vi "Check_Ch_Name_colons.vi"(1 "No of Colons":i32, 2 "Ch Name in":string) -> (0 "Ch Name out":string)   [LabVIEW 2018]
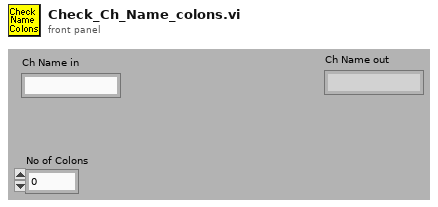
[diagram p1: front panel]
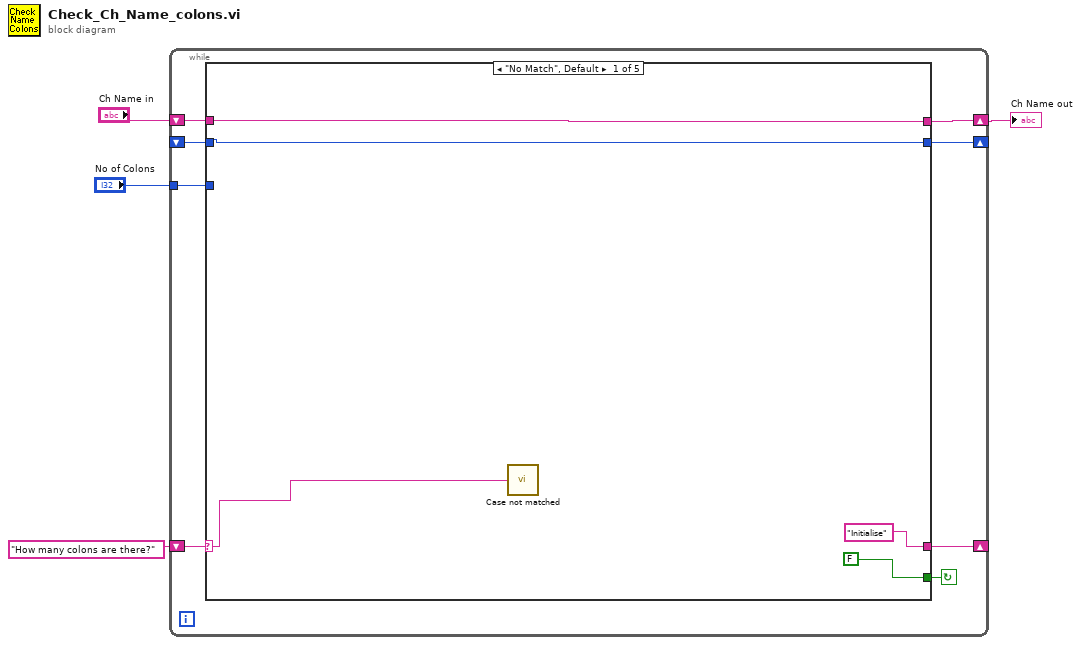
[diagram p0: block diagram]
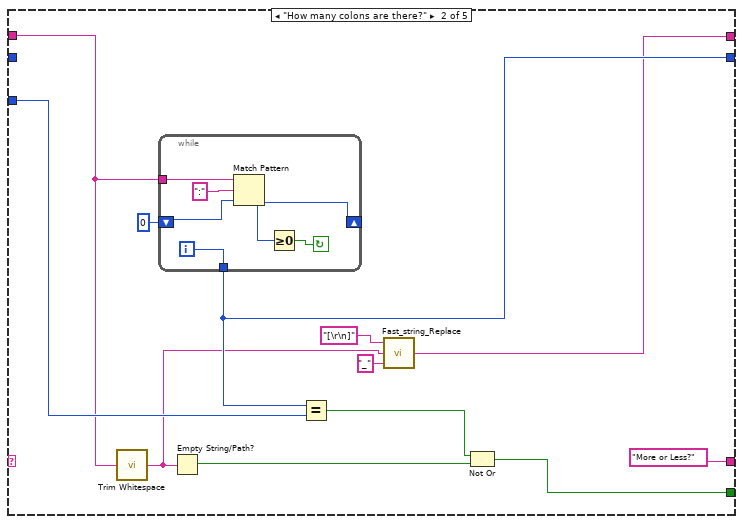
[diagram p2: hidden frame]
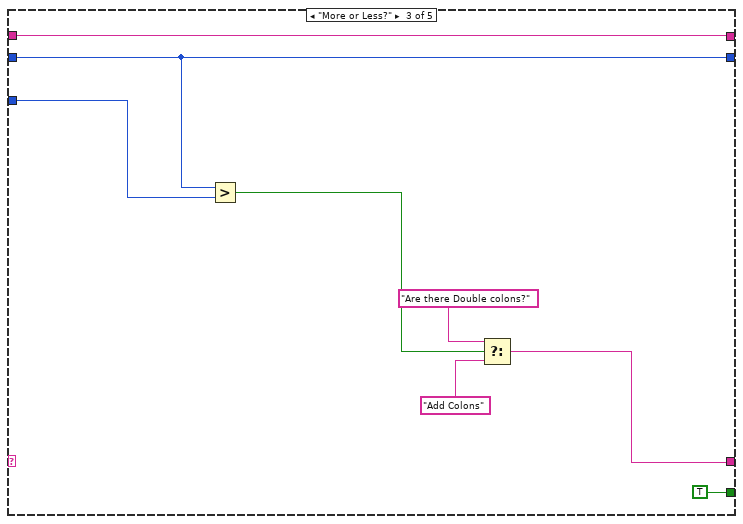
[diagram p3: hidden frame]
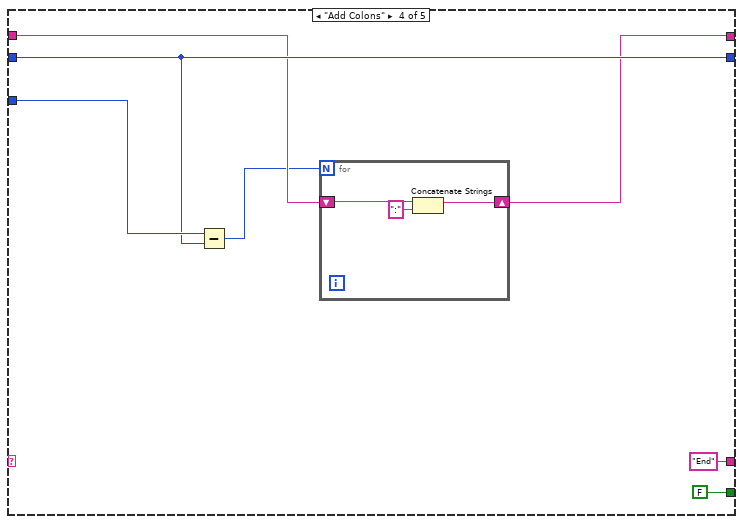
[diagram p4: hidden frame]
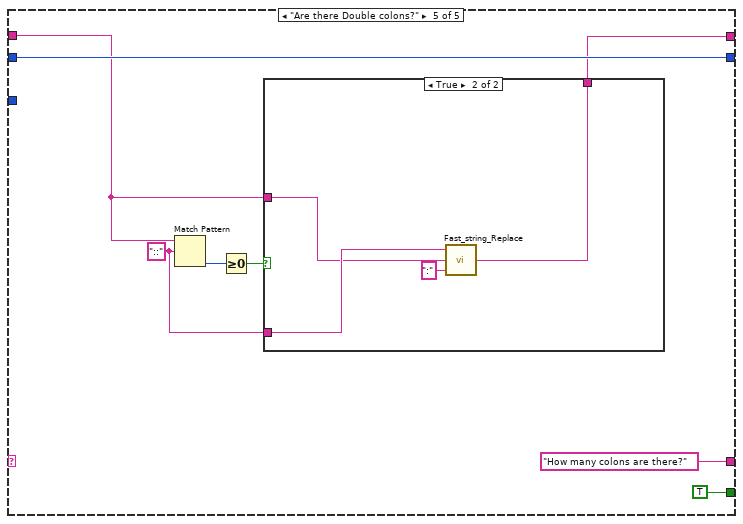
[diagram p5: hidden frame]
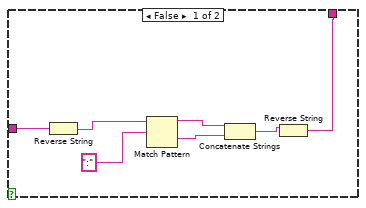
[diagram p6: hidden frame]
diagram:
  n1 = while {
    shift-left: "How many colons are there?" -> [w10]
    shift-right: [w11] -> _
    shift-right: [w8] -> w2
    shift-left: "Ch Name in" -> [w9]
    shift-right: [w7] -> _
    shift-left: _ -> [w6]
    tunnel: "No of Colons" -> [w5]
    stop <- w12 continue-if-true
    n2 = case shown="\"No Match\", Default" w10 {
      selector: w10 -> [w13 _ _ _ _]
      tunnel: [FALSE w23 TRUE FALSE TRUE] -> w12
      tunnel: ["Initialise" "More or Less?" w41 "End" "How many colons are there?"] -> w11
      tunnel: w9 -> [w15 w18 w38 w46 w55]
      tunnel: [w15 w20 w38 w47 w56] -> w8
      tunnel: w6 -> [w14 _ w37 w48 w60]
      tunnel: [w14 w27 w37 w48 w60] -> w7
      tunnel: w5 -> [_ w26 w43 w49 _]
      frame "No Match", Default {
        n3 = call "Case not matched.vi"("Case Name not Matched"=w13) -> ()
      }
      frame "How many colons are there?" {
        n4 = call <vilib>:"Trim Whitespace.vi"("string"=w18) -> ("trimmed string"=w21:string)  [unwired: 1 in]
        n5 = while {
          tunnel: w18 -> [w35]
          shift-right: [w31] -> _
          shift-left: 0 ("offset past match") -> [w33]
          tunnel: [w30] -> w27
          i -> [w30]
          stop <- w32 continue-if-true
          n6 = Match Pattern(string=w35, regular expression=":", offset (0)=w33) -> (offset past match=w31:i32)  [unwired: 3 out]
          n7 = Greater Or Equal To 0?(x=w31) -> (x >= 0?=w32:bool)
        }
        n8 = Empty String/Path?(string/path=w21) -> (empty?=w25:bool)
        n9 = Equal?(x=w27, y=w26) -> (x = y?=w24:bool)
        n10 = call "Fast_string_Replace.vi"("Replace match with:"="_", "Input String"=w21, "regular expression"="[\r\n]") -> ("Output String"=w20:string)  [unwired: 2 out]
        n11 = Not Or(1:w25, 2:w24) -> (0:w23:bool)
      }
      frame "More or Less?" {
        n12 = Greater?(x=w37, y=w43) -> (0:w42:bool)
        n13 = Select(t="Are there Double colons?", s=w42, f="Add Colons") -> (s? t:f=w41:string)
      }
      frame "Add Colons" {
        n14 = Subtract(x=w49, y=w48) -> (x-y=w45:i32)
        n15 = for {
          N: w45 -> [_]
          shift-right: [w51] -> w47
          shift-left: w46 -> [w53]
          n16 = Concatenate Strings(w53, ":" ("string")) -> (w51:string)
        }
      }
      frame "Are there Double colons?" {
        w57 = "::" ("regular expression")
        n17 = Match Pattern(string=w55, regular expression=w57) -> (offset past match=w59:i32)  [unwired: 4 out]
        n18 = Greater Or Equal To 0?(x=w59) -> (x >= 0?=w58:bool)
        n19 = case shown="True" w58 {
          tunnel: w57 -> [_ w72]
          tunnel: w55 -> [w68 w71]
          tunnel: [w62 w70] -> w56
          frame False {
            n20 = Reverse String(1:w68) -> (0:w66:string)
            n21 = Match Pattern(string=w66, regular expression=":") -> (before substring=w65:string, after substring=w64:string)  [unwired: 3 out]
            n22 = Concatenate Strings(w65, w64) -> (w63:string)
            n23 = Reverse String(1:w63) -> (0:w62:string)
          }
          frame True {
            n24 = call "Fast_string_Replace.vi"("Replace match with:"=":", "Input String"=w71, "regular expression"=w72) -> ("Output String"=w70:string)  [unwired: 2 out]
          }
        }
      }
    }
  }
  "Ch Name out" <- w2
